vi "b2w2.vi"(1 "parrel input":bool[](array[boolean]), 2 "bits-per-symbol":i32, 3 "number of subcarriers":i32) -> (0 "output array":bool[][](array[boolean]))   [LabVIEW 2013]
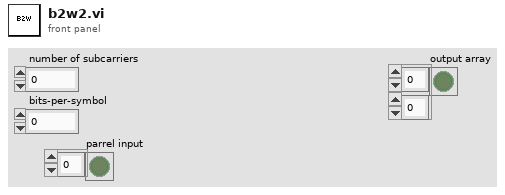
[diagram p1: front panel]
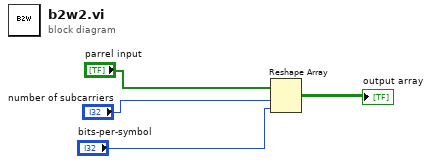
[diagram p0: block diagram]
diagram:
  n1 = Reshape Array("parrel input", "number of subcarriers", "bits-per-symbol") -> (→"output array":bool[][])
